vi "SingleLoopTemplate.Tester.vi"() -> ()   [LabVIEW 2025, in "ErrorViewer.lvclass"]
uses:
  ErrorViewer.lvclass
  ErrorViewer.lvclass/ErrorViewer.ctl
  C:/Git/JA/JQMH/RQMHCore/ModuleCore/RQMHModule.lvclass
  RQMHCore/ModuleCore/RQMHModule.lvclass
  RQMHCore/ModuleCore/Show Front Panel.vi
  RQMHCore/ModuleCore/Show In Subpanel.vi
panel:
  out "Last Error Time":timestamp
  out "last error":errorcluster
  out "Status":string
  in  "Tab Control":enum32{"Admin", "Commands"}(tab)
  in  "Exit":bool
  in  "Stop Module":bool
  in  "Show Block Diagram":bool
  in  "Hide Module Panel":bool
  in  "Show Module Panel":bool
  in  "Start Module":bool
  in  "Hide Block Diagram":bool
  in  "Show In SP":bool
  out "Launch Time (S)":dbl
  in  "Do Something":bool
  in  "Msg":string
  out "Value":dbl
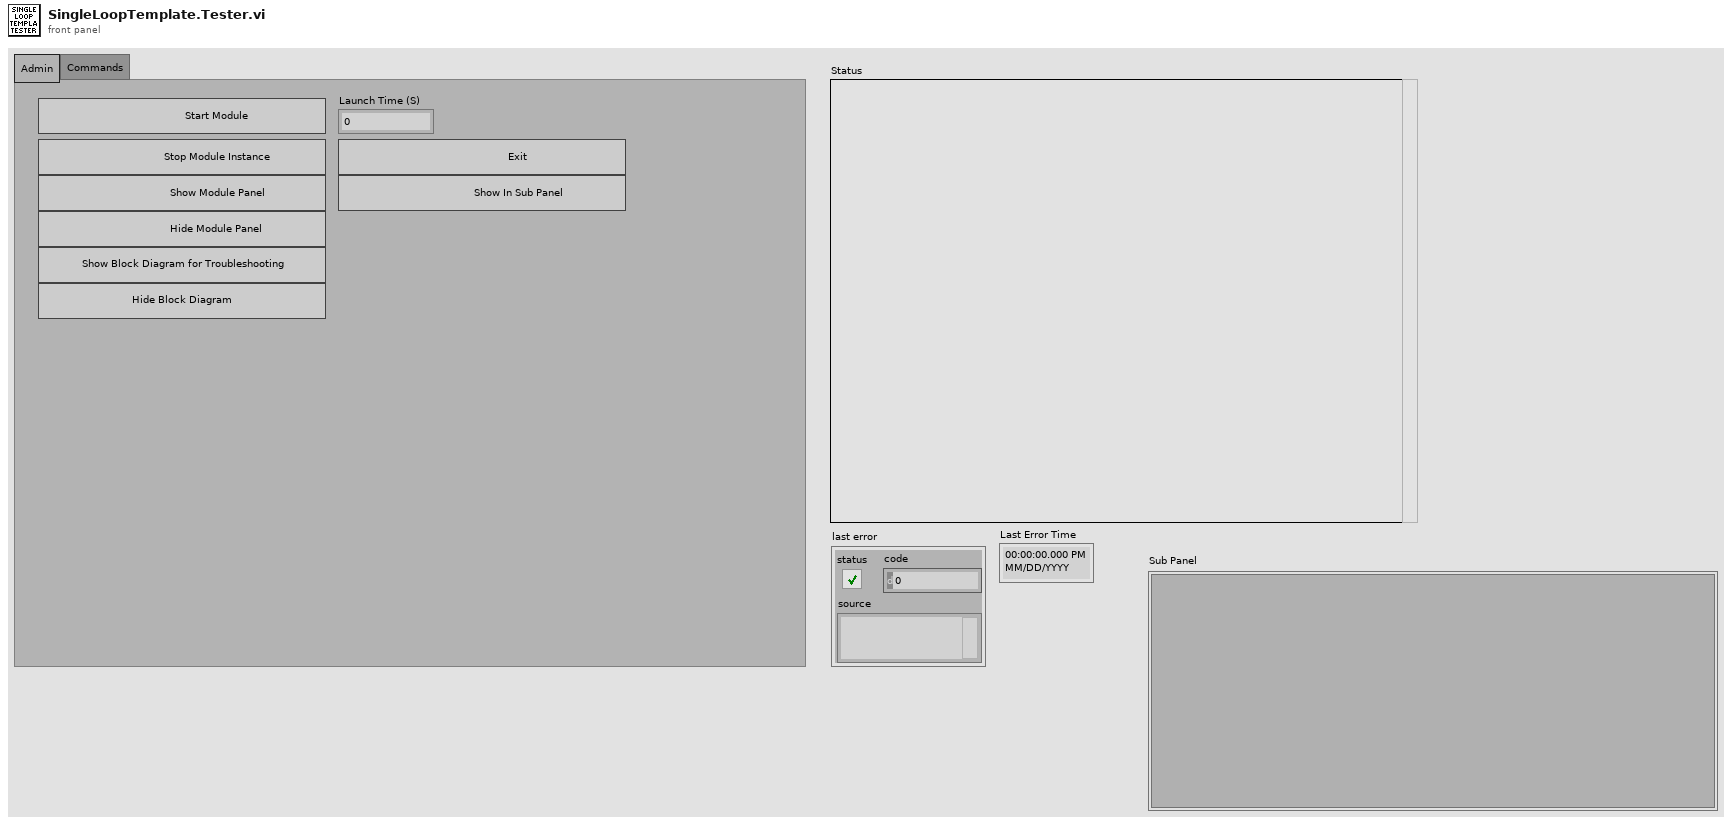
[diagram p1: front panel]
types:
  T1 = typedef "RQMHModule.lvclass/StandardBroadcasts.ctl" = cluster{"Died":refnum<user-event>, "Started":refnum<user-event>}
  T2 = typedef "ErrorViewer.lvclass/Broadcast Events--cluster.ctl" = cluster{"Stopped":refnum<user-event>}
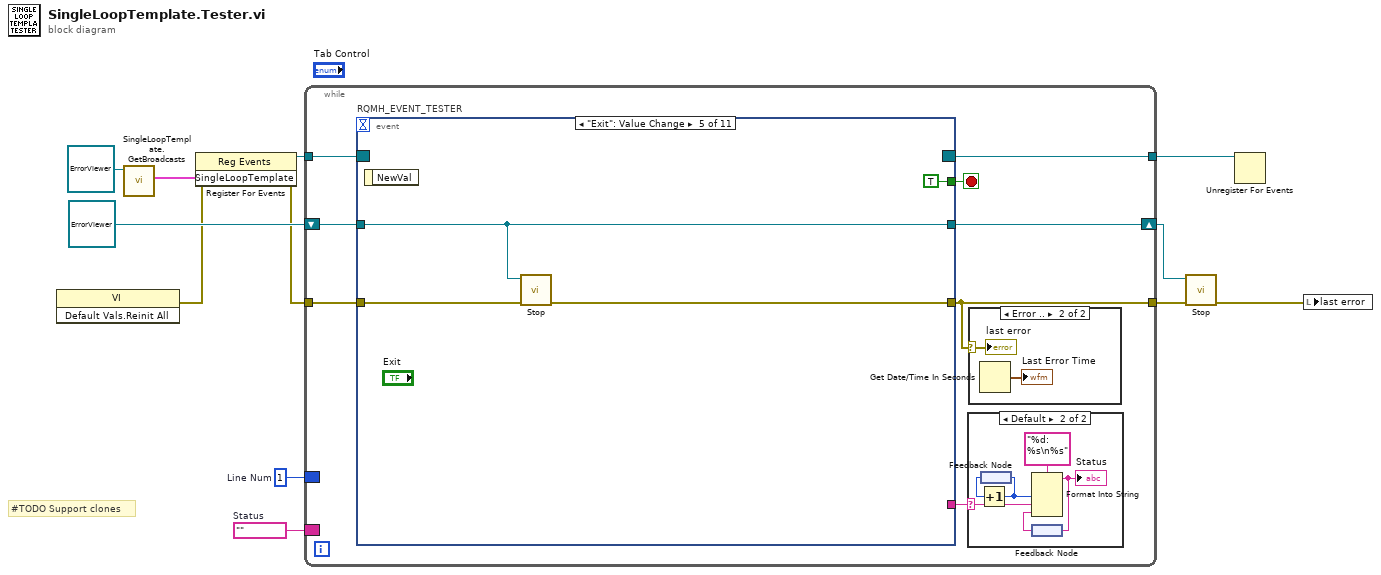
[diagram p0: block diagram]
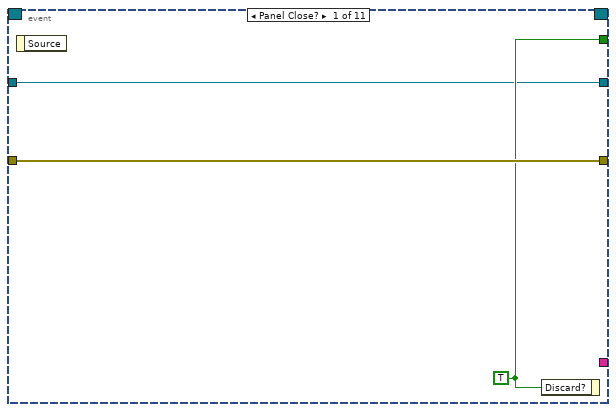
[diagram p2: hidden frame]
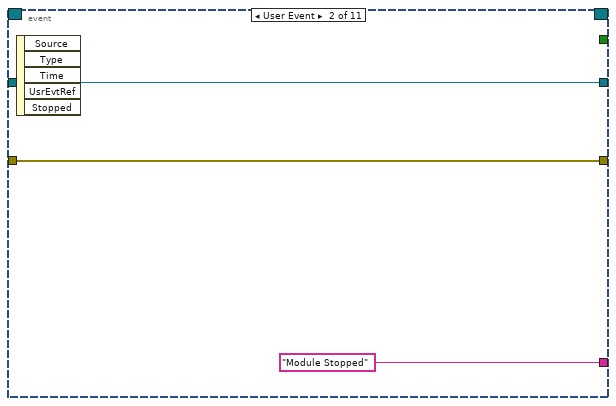
[diagram p3: hidden frame]
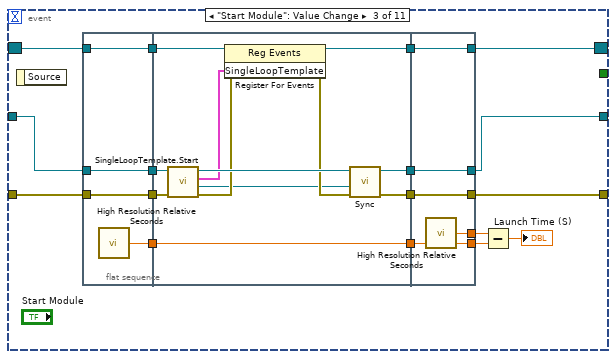
[diagram p4: hidden frame]
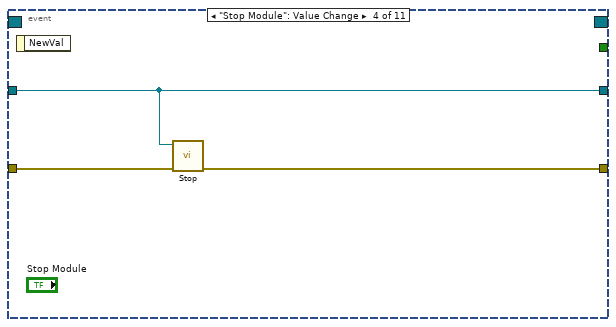
[diagram p5: hidden frame]
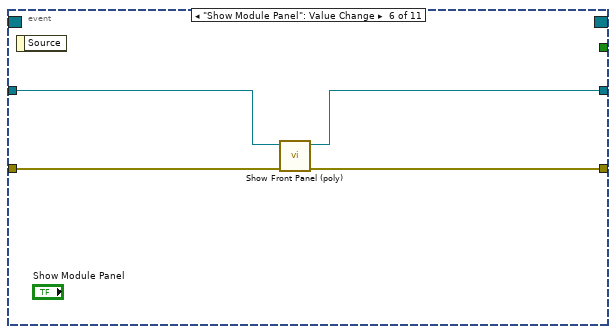
[diagram p6: hidden frame]
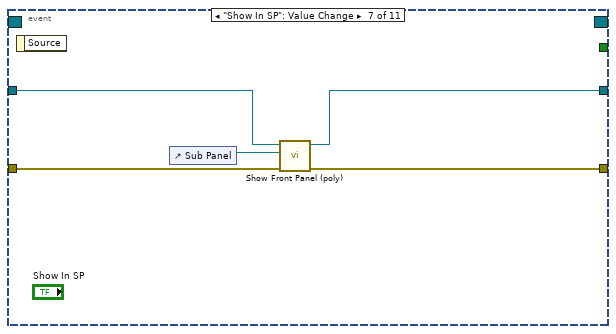
[diagram p7: hidden frame]
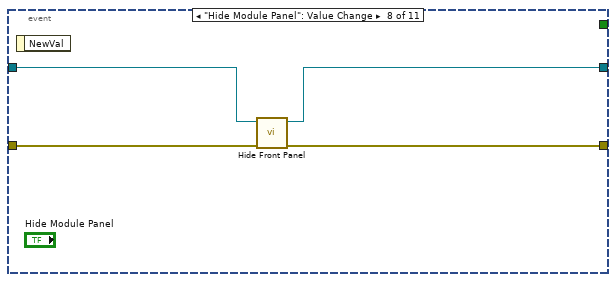
[diagram p8: hidden frame]
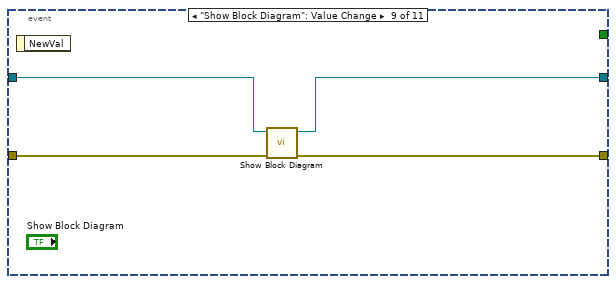
[diagram p9: hidden frame]
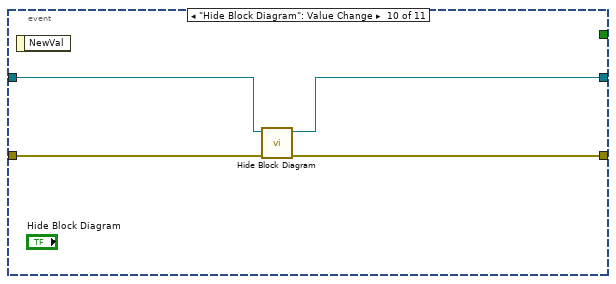
[diagram p10: hidden frame]
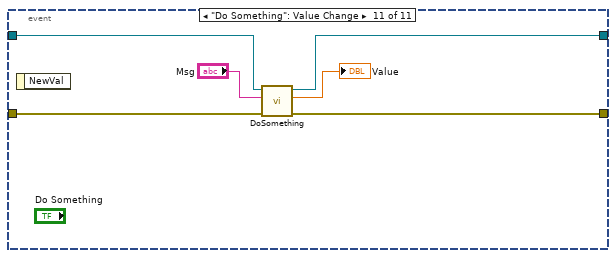
[diagram p11: hidden frame]
diagram:
  w1 = ""  # Status
  w2 = 1  # Line Num
  # "#TODO Support clones"
  n1 = invoke class="VI" method="Default Vals.Reinit All"() -> (error out=w7:errorcluster)  [unwired: 3 in, 2 out]
  n2 = call "SingleLoopTemplate.GetBroadcasts.vi"("NewTemplate in"=refnum<class "ErrorViewer.lvclass"> refnum ("TemplateModule in")) -> ("SingleLoopTemplate"=w11:cluster{"Broadcasts":T1, "Broadcasts":T2})  [unwired: 9 in, 1 out]
  n3 = register-events(error in=w7, w11) -> (reference out=w10:refnum<event-registration>, error out=w6:errorcluster)  [unwired: 1 in]
  n4 = while {
    tunnel: w6 -> [w19]
    tunnel: w10 -> [w20]
    tunnel: [w18] -> w4
    tunnel: [w16] -> w9
    shift-right: [w14] -> w5
    shift-left: refnum<class "ErrorViewer.lvclass"> refnum ("TemplateModule in") -> [w15]
    border: w2 -> [_]
    border: w1 -> [_]
    stop <- w17 stop-if-true
    n5 = event "RQMH_EVENT_TESTER" shown="[4] \"Exit\": Value Change" {
      selector: w20 -> [_ _ w41 _ _ _ _ _ _ _ _]
      dyn-events: [_ _ w40 _ _ _ _ _ _ _ _] -> w16
      timeout: _ -> [_ _ _ _ _ _ _ _ _ _ _]
      tunnel: w19 -> [w23 w26 w43 w67 w71 w74 w79 w83 w87 w91 w97]
      tunnel: [w23 w26 w39 w66 w70 w75 w80 w84 w88 w89 w95] -> w18
      tunnel: [w22 _ _ _ TRUE _ _ _ _ _ _] -> w17
      tunnel: w15 -> [w21 w25 w42 w65 w69 w72 w77 w81 w85 w92 w98]
      tunnel: [w21 w25 w38 w65 w69 w73 w78 w82 w86 w90 w96] -> w14
      tunnel: [_ "Module Stopped" _ _ _ _ _ _ _ _ _] -> w13
      event Panel Close? {
        w22 = TRUE
        n6 = event-data() -> ()  [unwired: 1 in, 1 out]
        n7 = event-data("Discard?"=w22) -> ()  [unwired: 1 in, 1 out]
      }
      event User Event {
        n8 = event-data() -> ()  [unwired: 1 in, 5 out]
      }
      event "Start Module": Value Change {
        n9 = event-data() -> ()  [unwired: 1 in, 1 out]
        n10 = flat-sequence {
          tunnel: w41 -> [w45]
          tunnel: w42 -> [w46]
          tunnel: w43 -> [w47]
          tunnel: [w47] -> w37
          tunnel: [w46] -> w36
          tunnel: [w45] -> w35
          tunnel: [w44] -> w28
          tunnel: w37 -> [w59]
          tunnel: w36 -> [w58]
          tunnel: w35 -> [w57]
          tunnel: [w56] -> w34
          tunnel: [w55] -> w33
          tunnel: [w50] -> w32
          tunnel: [w48] -> w29
          tunnel: w28 -> [w48]
          tunnel: [w62] -> w38
          tunnel: [w63] -> w39
          tunnel: [w64] -> w40
          tunnel: w34 -> [w64]
          tunnel: w33 -> [w63]
          tunnel: w32 -> [w62]
          tunnel: [w61] -> w31
          tunnel: [w60] -> w30
          tunnel: w29 -> [w60]
          frame #0 {
            n11 = call <vilib>:"High Resolution Relative Seconds.vi"() -> ("relative seconds"=w44:dbl)
          }
          frame #1 {
            n12 = call "SingleLoopTemplate.Start.vi"("error in (no error)"=w59, "NewTemplate in"=w58) -> ("error out"=w53:errorcluster, "StartupHandshake out"=w51:refnum<class "RQMHStartup.lvclass">, "_TemplateModule"=w49:cluster{"Broadcasts":T1, "Broadcasts":T2}, "NewTemplate out"=w54:refnum<class "ErrorViewer.lvclass">)  [unwired: 6 in]
            n13 = register-events(reference=w57, error in=w53, w49) -> (reference out=w56:refnum<event-registration>, error out=w52:errorcluster)
            n14 = call "Sync.vi"("error in (no error)"=w52, "StartupHandshake out"=w51, "JQMHCore in"=w54) -> ("error out"=w55:errorcluster, "JQMHCore out"=w50:refnum<class "ErrorViewer.lvclass">)  [unwired: 7 in]
          }
          frame #2 {
            n15 = call <vilib>:"High Resolution Relative Seconds.vi"() -> ("relative seconds"=w61:dbl)
          }
        }
        n16 = Subtract(x=w31, y=w30) -> (x-y=→"Launch Time (S)":dbl)
      }
      event "Stop Module": Value Change {
        n17 = event-data() -> ()  [unwired: 1 in, 1 out]
        n18 = call "Stop.vi"("error in (no error)"=w67, "JQMHCore in"=w65) -> ("error out"=w66:errorcluster)  [unwired: 9 in]
      }
      event "Exit": Value Change {
        n19 = event-data() -> ()  [unwired: 1 in, 1 out]
        n20 = call "Stop.vi"("error in (no error)"=w71, "JQMHCore in"=w69) -> ("error out"=w70:errorcluster)  [unwired: 9 in]
      }
      event "Show Module Panel": Value Change {
        n21 = event-data() -> ()  [unwired: 1 in, 1 out]
        n22 = call-poly "Show Front Panel (poly).vi"("error in (no error)"=w74, "JQMHCore in"=w72) -> ("error out"=w75:errorcluster, "JQMHCore in"=w73:refnum<class "ErrorViewer.lvclass">)  [unwired: 8 in]
      }
      event "Show In SP": Value Change {
        n23 = event-data() -> ()  [unwired: 1 in, 1 out]
        n24 = control-ref of="Sub Panel"() -> (w76:refnum<vi>)
        n25 = call-poly "Show Front Panel (poly).vi"("error in (no error)"=w79, "Sub Panel"=w76, "JQMHCore in"=w77) -> ("error out"=w80:errorcluster, "JQMHCore in"=w78:refnum<class "ErrorViewer.lvclass">)  [unwired: 7 in]
      }
      event "Hide Module Panel": Value Change {
        n26 = event-data() -> ()  [unwired: 1 in, 1 out]
        n27 = call "Hide Front Panel.vi"("error in (no error)"=w83, "JQMHCore in"=w81) -> ("error out"=w84:errorcluster, "JQMHCore in"=w82:refnum<class "ErrorViewer.lvclass">)  [unwired: 8 in]
      }
      event "Show Block Diagram": Value Change {
        n28 = event-data() -> ()  [unwired: 1 in, 1 out]
        n29 = call "Show Block Diagram.vi"("error in (no error)"=w87, "JQMHCore in"=w85) -> ("error out"=w88:errorcluster, "JQMHCore in"=w86:refnum<class "ErrorViewer.lvclass">)  [unwired: 8 in]
      }
      event "Hide Block Diagram": Value Change {
        n30 = event-data() -> ()  [unwired: 1 in, 1 out]
        n31 = call "Hide Block Diagram.vi"("error in (no error)"=w91, "JQMHCore in"=w92) -> ("error out"=w89:errorcluster, "JQMHCore in"=w90:refnum<class "ErrorViewer.lvclass">)  [unwired: 8 in]
      }
      event "Do Something": Value Change {
        n32 = event-data() -> ()  [unwired: 1 in, 1 out]
        n33 = call "DoSomething.vi"("error in (no error)"=w97, "Msg"="Msg", "NewTemplate in"=w98) -> ("error out"=w95:errorcluster, "Value"=→"Value":dbl, "NewTemplate out"=w96:refnum<class "ErrorViewer.lvclass">)  [unwired: 5 in, 1 out]
      }
    }
    n34 = case "RQMH_TESTER_STATUS" shown="Default" w13 {
      selector: w13 -> [_ w102]
      frame "" {
      }
      frame Default {
        n35 = feedback #1() -> (w101:i32)
        n36 = Increment(x=w101) -> (x+1=w100:i32)
        n37 = feedback-in #1(w100) -> ()
        n38 = feedback #2() -> (w103:string)
        n39 = Format Into String(format string="%d: %s\n%s", w100, w102, w103) -> (resulting string=w99:string)  [unwired: 2 in, 1 out]
        "Status" <- w99
        n40 = feedback-in #2(w99) -> ()
      }
    }
    n41 = case shown="Error .." w18 {
      selector: w18 -> [_ w106]
      frame No Error {
      }
      frame Error {
        n42 = Get Date/Time In Seconds() -> (seconds since 1Jan1904=→"Last Error Time":timestamp)
        "last error" <- w106
      }
    }
  }
  n43 = call "Stop.vi"("error in (no error)"=w4, "JQMHCore in"=w5) -> ("error out"=w3:errorcluster)  [unwired: 9 in]
  n44 = Unregister For Events(event registration refnum=w9) -> ()  [unwired: 1 in, 1 out]
  n45 = local write "last error"(w3) -> ()
